vi "ErrorMessageBuilder.vi"(3 "Error Triggers":bool[](array[boolean]), 4 "Delays (s)":dbl[](array[numeric]), 5 "Error Messages":string[](array[string])) -> (1 "Combined Error String":string)   [LabVIEW 2018]
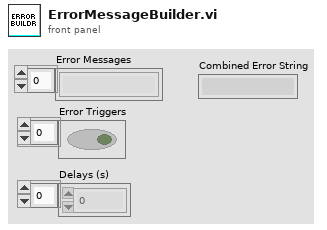
[diagram p1: front panel]
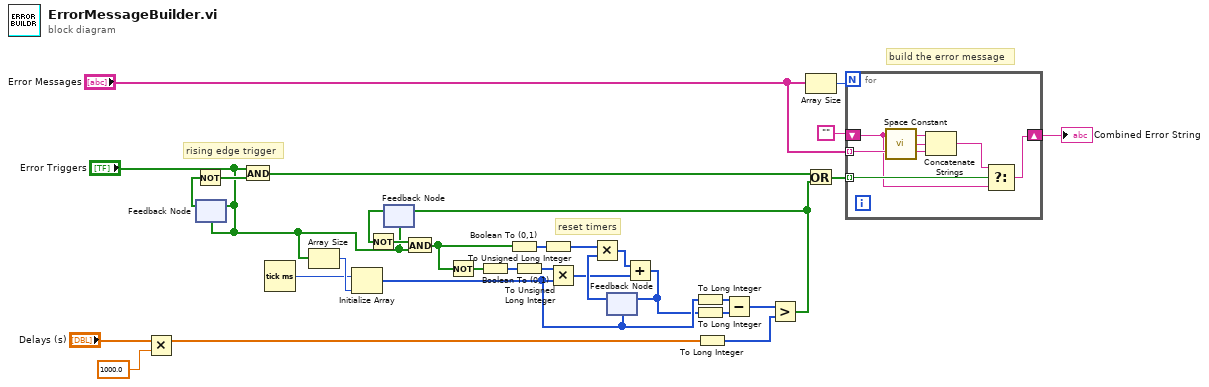
[diagram p0: block diagram]
diagram:
  # "build the error message"
  # "reset timers"
  # "rising edge trigger"
  n1 = Multiply(x="Delays (s)", y=1000.0) -> (x*y=w3:dbl[])
  n2 = feedback #1("Error Triggers") -> (w7:bool[])
  n3 = Not(x=w7) -> (.not. x?=w25:bool[])
  n4 = feedback-in #1("Error Triggers") -> ()
  n5 = And(x="Error Triggers", y=w25) -> (x .and. y?=w31:bool[])
  n6 = Tick Count (ms)() -> (millisecond timer value=w10:u32)
  n7 = Array Size(array="Error Triggers") -> (size(s)=w23:i32)
  n8 = Initialize Array(w10, w23) -> (w21:u32[])
  n9 = feedback #2("Error Triggers") -> (w28:bool[])
  n10 = Not(x=w28) -> (.not. x?=w29:bool[])
  n11 = And(x=w29, y="Error Triggers") -> (x .and. y?=w27:bool[])
  n12 = Not(x=w27) -> (.not. x?=w26:bool[])
  n13 = Boolean To (0,1)(Boolean=w26) -> (0, 1=w11:i16[])
  n14 = Boolean To (0,1)(Boolean=w27) -> (0, 1=w13:i16[])
  n15 = To Unsigned Long Integer(number=w11) -> (unsigned 32bit integer=w12:u32[])
  n16 = To Unsigned Long Integer(number=w13) -> (unsigned 32bit integer=w15:u32[])
  n17 = Multiply(x=w12, y=w21) -> (x*y=w14:u32[])
  n18 = feedback #3(w21) -> (w16:u32[])
  n19 = Multiply(x=w15, y=w16) -> (x*y=w17:u32[])
  n20 = Add(x=w17, y=w14) -> (x+y=w20:u32[])
  n21 = feedback-in #3(w20) -> ()
  n22 = To Long Integer(number=w21) -> (32bit integer=w18:i32[])
  n23 = To Long Integer(number=w20) -> (32bit integer=w19:i32[])
  n24 = To Long Integer(number=w3) -> (32bit integer=w24:i32[])
  n25 = Subtract(x=w18, y=w19) -> (x-y=w22:i32[])
  n26 = Greater?(x=w22, y=w24) -> (0:w30:bool[])
  n27 = feedback-in #2(w30) -> ()
  n28 = Array Size(array="Error Messages") -> (size(s)=w6:i32)
  n29 = Or(x=w31, y=w30) -> (x .or. y?=w32:bool[])
  n30 = for {
    N: w6 -> [_]
    tunnel: w32 -> [w38] mode=indexing
    tunnel: "Error Messages" -> [w36] mode=indexing
    shift-right: [w34] -> w8
    shift-left: "" -> [w33]
    n31 = call <vilib>:"Space Constant.vi"() -> ("String"=w37:string)
    n32 = Concatenate Strings(w33, w37, w36) -> (w35:string)
    n33 = Select(t=w35, s=w38, f=w33) -> (s? t:f=w34:string)
  }
  "Combined Error String" <- w8
